vi "Error Handler.vi"(7 "Actor in":refnum<class "Actor.lvclass">, 8 "Error in":errorcluster, 10 "From Msg Event":bool) -> (0 "Error out":errorcluster, 2 "Stop":bool, 5 "Actor out":refnum<class "Actor.lvclass">)   [LabVIEW 2025, in "jettl.lvlib" / "Actor.lvlib"]
uses:
  Actor.lvlib
  Actor/Actor.lvclass
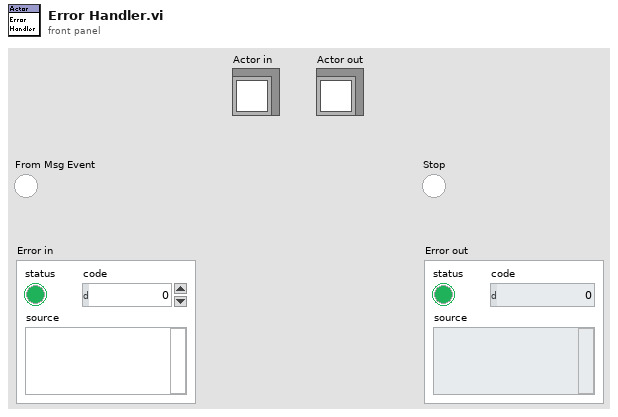
[diagram p1: front panel]
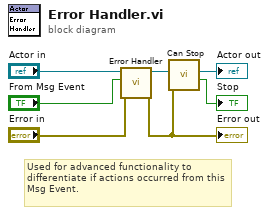
[diagram p0: block diagram]
diagram:
  # "Used for advanced functionality to differentiate if actions occurred from this Msg Event."
  n1 = call-dynamic "Error Handler.vi"("Error in"="Error in", "From Msg Event"="From Msg Event", "Actor in"="Actor in") -> ("Error out"=w6:errorcluster, "Actor out"=w7:refnum<class "Actor.lvclass">)  [unwired: 7 in]
  "Error out" <- w6
  n2 = call "Can Stop.vi"("Error in"=w6, "Actor in"=w7) -> ("Stop"=→"Stop":bool, "Actor out"=→"Actor out":refnum<class "Actor.lvclass">)  [unwired: 8 in]
